vi "gen MB frame -Set the device address.vi"(11 "Dev Addr":u8=1) -> (3 "MB frame":string)   [LabVIEW 2016, in "MB _relays.lvlib"]
uses:
  MB _relays.lvlib
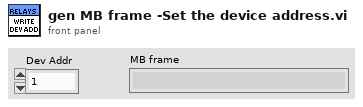
[diagram p1: front panel]
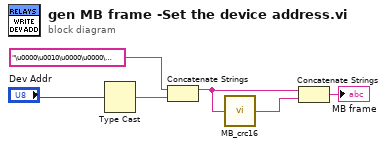
[diagram p0: block diagram]
diagram:
  n1 = Type Cast(x="Dev Addr") -> (*(type *) &x=w2:string)  [unwired: 1 in]
  n2 = Concatenate Strings("\u0000\u0010\u0000\u0000\u0000\u0001\u0002\u0000", w2) -> (w5:string)
  n3 = call "MB_crc16.vi"("message"=w5) -> ("CRC16"=w4:string)  [unwired: 4 in]
  n4 = Concatenate Strings(w5, w4) -> (→"MB frame":string)
